vi "Integer.vi"() -> (0 "error out":errorcluster, 3 "Passed?":bool)   [LabVIEW 2009]
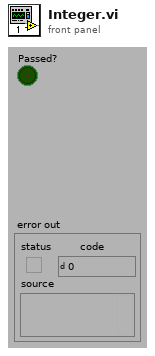
[diagram p1: front panel]
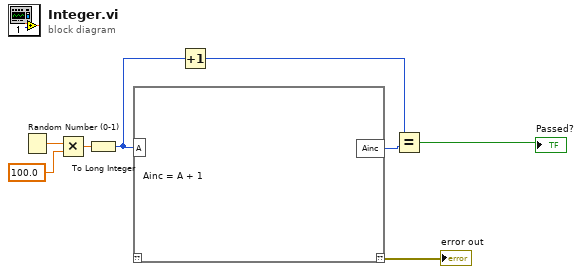
[diagram p0: block diagram]
diagram:
  n1 = Random Number (0-1)() -> (number: 0 to 1=w7:dbl)
  n2 = Multiply(x=w7, y=100.0) -> (x*y=w5:dbl)
  n3 = To Long Integer(number=w5) -> (32bit integer=w4:i32)
  n4 = script code="Ainc = A + 1"("A"=w4) -> ("??"=→"error out":errorcluster, "Ainc"=w3:i32)  [unwired: 1 in]
  n5 = Increment(x=w4) -> (x+1=w2:i32)
  n6 = Equal?(x=w2, y=w3) -> (x = y?=→"Passed?":bool)
